vi "Test Save JPG (Path).vi"(8 "error in (no error)":errorcluster) -> (0 "error out":errorcluster, 3 "Pass?":bool)   [LabVIEW 2020]
uses:
  <vilib>/picture/picture.llb/imagedata.ctl
  G-Image/Image IO/Polymorphic VIs/Load Image (Path).vi
  G-Image/G-Image.lvlib
  G-Image/Image IO/Polymorphic VIs/Save JPG Image (Path).vi
panel:
  out "Array":cluster{string, "new picture":picture}[](array[cluster])
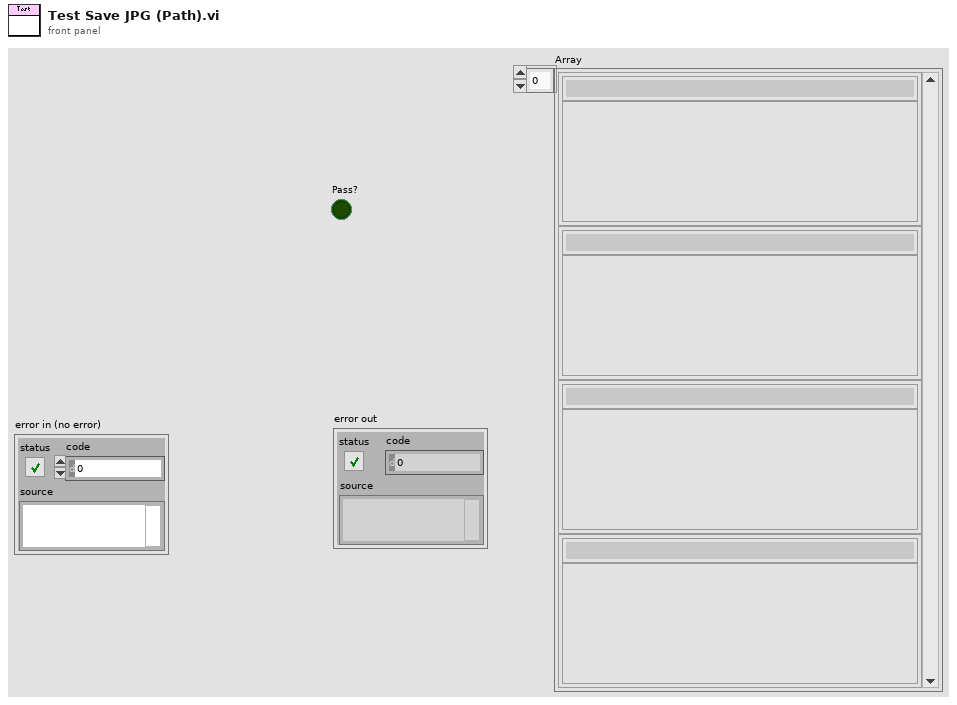
[diagram p1: front panel]
types:
  T1 = typedef "imagedata.ctl" = cluster{"image type":i32, "image depth":i32, "image":u8[], "mask":u8[], "colors":u32[], "Rectangle":cluster{"left":i16, "top":i16, "right":i16, "bottom":i16}}
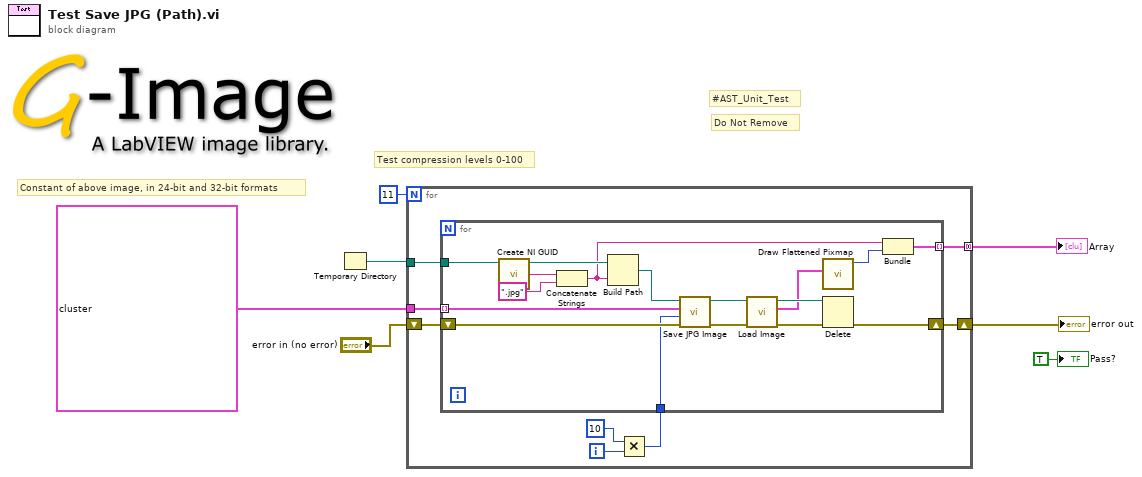
[diagram p0: block diagram]
diagram:
  # "Test compression levels 0-100"
  # "Constant of above image, in 24-bit and 32-bit formats"
  # "Do Not Remove"
  # "#AST_Unit_Test"
  n1 = Temporary Directory() -> (w6:path)
  n2 = for {
    N: 11 -> [_]
    tunnel: w6 -> [w14]
    tunnel: [w13] -> w5 mode=concatenating
    tunnel: T1[] [{"image type"=0, "image depth"=24, "image"=array[115500 elements], "mask"=[], "colors"=[], "Rectangle"={"left"=0, "top"=0, "right"=350, "bottom"=110}}, {"image type"=0, "image depth"=32, "image"=array[154000 elements], "mask"=array[4840 elements], "colors"=[], "Rectangle"={"left"=0, "top"=0, "right"=350, "bottom"=110}}] ("Array 2") -> [w11]
    shift-right: [w12] -> w4
    shift-left: "error in (no error)" -> [w15]
    i -> [w10]
    n3 = Multiply(x=10, y=w10) -> (x*y=w8:i32)
    n4 = for {
      tunnel: w14 -> [w28]
      tunnel: w11 -> [w24] mode=indexing
      shift-right: [w21] -> w12
      shift-left: w15 -> [w31]
      tunnel: [w17] -> w13 mode=indexing
      tunnel: w8 -> [w16]
      n5 = call <vilib>:"Create NI GUID.vi"() -> ("NI GUID"=w29:string)
      n6 = Concatenate Strings(w29, ".jpg" ("string")) -> (w18:string)
      n7 = Build Path(base path=w28, name or relative path=w18) -> (appended path=w27:path)
      n8 = call-poly "Save JPG Image.vi"("error in (no error)"=w31, "Quality (85)"=w16, "Image"=w24, "Path In"=w27) -> ("error out"=w25:errorcluster, "Path Out"=w26:path)  [unwired: 6 in]
      n9 = call-poly "Load Image.vi"("error in (no error)"=w25, "Path In"=w26) -> ("error out"=w22:errorcluster, "Image"=w20:T1, "Path Out"=w23:path)  [unwired: 7 in]
      n10 = call <vilib>:"Draw Flattened Pixmap.vi"("image data"=w20) -> ("new picture"=w19:picture)  [unwired: 8 in]
      n11 = Delete(path (use dialog)=w23, error in=w22) -> (error out=w21:errorcluster)  [unwired: 3 in, 2 out]
      n12 = Bundle(w18, "new picture"=w19) -> (w17:cluster{string, "new picture":picture})  [unwired: 1 in]
    }
  }
  "error out" <- w4
  "Array" <- w5
  "Pass?" <- TRUE ("Pass?")
